vi "Remove APU.vi"(8 "error in (no error)":errorcluster, 11 "APU":refnum<k24>) -> (0 "error out":errorcluster)   [LabVIEW 2020, in "Engine Simulation Toolkit Scripting API.lvlib"]
uses:
  Engine Simulation Toolkit Scripting API.lvlib
  NationalInstruments.VeriStand.SystemDefinitionAPI
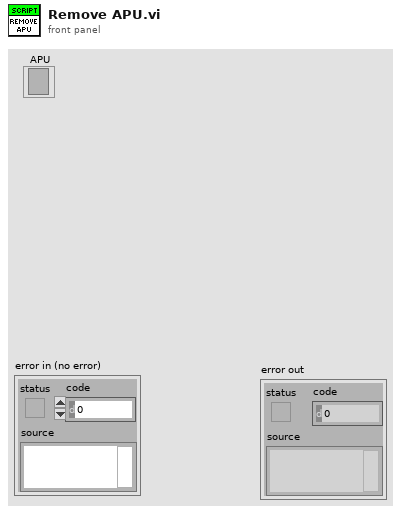
[diagram p1: front panel]
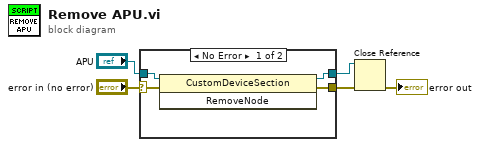
[diagram p0: block diagram]
diagram:
  n1 = case shown="No Error" "error in (no error)" {
    selector: "error in (no error)" -> [w8 w11]
    tunnel: [w7 w11] -> w2
    tunnel: "APU" -> [w9 w10]
    tunnel: [w6 w10] -> w3
    frame No Error {
      n2 = invoke class="CustomDeviceSection" method="RemoveNode"(reference=w9, error in=w8) -> (reference out=w6:refnum<k24>, error out=w7:errorcluster)  [unwired: 1 in, 1 out]
    }
    frame Error {
    }
  }
  n3 = Close Reference(reference=w3, error in (no error)=w2) -> (error out=→"error out":errorcluster)
